vi "VisionPositionControlAngleToSpeaker.vi"() -> ()   [LabVIEW 2023]
doc: "Position control for angle to speaker\ninputs:\n--TargetPosition--degrees--Numeric--(probably use VisionGetDistanceAndAngleToSpeaker)\noutputs:\n--DesiredSpeed--degrees/s--Numeric\n--OnTarget--boolean"
uses:
  <vilib>/Rock Robotics/WPI/ThirdParty/JAS_Junk/TrajLib/Trajectory_Library.lvlib
panel:
  in  "TargetPosition":dbl
  out "OnTarget":bool
  out "DesiredSpeed (degree/s)":dbl
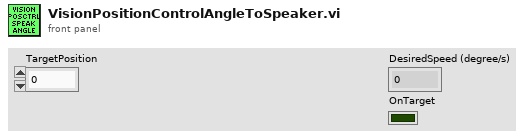
[diagram p1: front panel]
types:
  T1 = typedef "Trajectory_Library.lvlib/POSE2D.ctl" = cluster{"TRANSLATION":T2, "ROTATION":T3}
  T2 = typedef "Trajectory_Library.lvlib/TRANSLATION2D.ctl" = cluster{"X":dbl, "Y":dbl}
  T3 = typedef "Trajectory_Library.lvlib/ROTATION2D.ctl" = cluster{"VALUE":dbl, "COS":dbl, "SIN":dbl}
  T4 = typedef "Trajectory_Library.lvlib/PosCtrl_Tuning_Type.ctl" = cluster{"Slope":dbl, "Offset":dbl, "Error Deadband":dbl, "At Reference Count":i32, "Negate Output":bool, "Max Allowd Position":dbl, "Min Allowd Position":dbl}
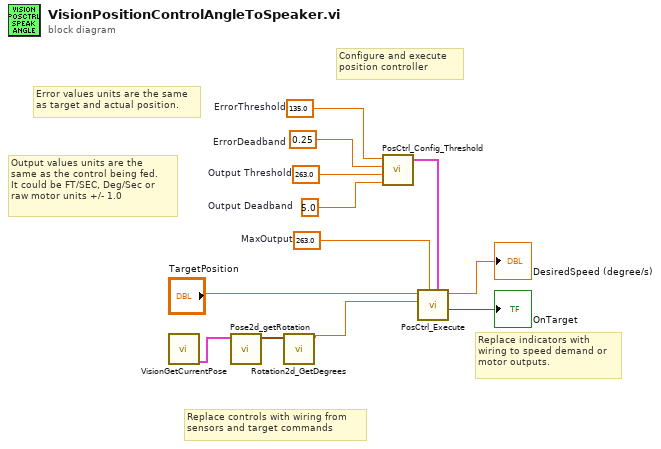
[diagram p0: block diagram]
diagram:
  w12 = 263.0  # MaxOutput
  w8 = 135.0  # ErrorThreshold
  w7 = 0.25  # ErrorDeadband
  w6 = 263.0  # Output Threshold
  w5 = 5.0  # Output Deadband
  # "Replace controls with wiring from\nsensors and target commands"
  # "Replace indicators with\nwiring to speed demand or\nmotor outputs."
  # "Output values units are the\nsame as the control being fed.  \nIt could be FT/SEC, Deg/Sec or\nraw motor units +/- 1.0"
  # "Error values units are the same \nas target and actual position."
  # "Configure and execute \nposition controller"
  n1 = call "VisionGetCurrentPose.vi"() -> ("Current Pose"=w1:T1)  [unwired: 9 in]
  n2 = call <vilib>:"Pose2d_getRotation.vi"("in POSE"=w1) -> ("out ROTATION"=w3:T3)  [unwired: 10 in]
  n3 = call <vilib>:"Rotation2d_GetDegrees.vi"("in ROTATION"=w3) -> ("AngleDegrees"=w2:dbl)  [unwired: 10 in]
  n4 = call <vilib>:"PosCtrl_Config_Threshold.vi"("Output Deadband"=w5, "Output Threshold"=w6, "ErrorDeadband"=w7, "ErrorThreshold"=w8) -> ("PosCtrl_Config_Params"=w9:T4)  [unwired: 7 in]
  n5 = call <vilib>:"PosCtrl_Execute.vi"("PosCtrl_Config_Params"=w9, "MaxOutput"=w12, "CurrentPosition"=w2, "TargetPosition"="TargetPosition") -> ("OnTarget"=→"OnTarget":bool, "Output"=→"DesiredSpeed (degree/s)":dbl)  [unwired: 5 in, 1 out]
